vi "Fetch Multi Eval Meas Power Dynamics Results.vi"(8 "error in (no error)":errorcluster, 9 "Result Type (Current)":i32(ring) items=["Current"=0, "Average"=1, "Standard Deviation"=3, "Maximum"=4, "Minimum"=5], 10 "Instance (1)":T2=1, 11 "VISA resource name":refnum<visa-resource-name>) -> (0 "error out":errorcluster, 1 "Results":T1 {"Off Power After" format="%^.3e"; "On Power Peak" format="%^.3e"; "On Power RMS" format="%^.3e"; "Off Power Before" format="%^.3e"}, 2 "Reliability":i32, 3 "VISA resource name out":refnum<visa-resource-name>, 4 "Out Of Tolerance":dbl format="%^.3e")   [LabVIEW 2015, in "Rohde&Schwarz CMXP NR FR2 Measurement.lvlib"]
doc: "Returns the average single value results of the power dynamics measurement.\n\nAttributes:\nRSCMXPNRFR2M_ATTR_FETCH_MULTI_EVAL_MEASUREMENT_POWER_DYNAMICS_AVERAGE_RESULTS\nRSCMXPNRFR2M_ATTR_FETCH_MULTI_EVAL_MEASUREMENT_POWER_DYNAMICS_CURRENT_RESULTS\nRSCMXPNRFR2M_ATTR_FETCH_MULTI_EVAL_MEASUREMENT_POWER_DYNAMICS_MAXIMUM_RESULTS\nRSCMXPNRFR2M_ATTR_FETCH_MULTI_EVAL_MEASUREMENT_POWER_DYNAMICS_MINIMUM_RESULTS\nRSCMXPNRFR2M_ATTR_FETCH_MULTI_EVAL_MEASUREMENT_POWER_DYNAMICS_STANDARD_DEVIATION_RESULTS\n\nRemote-control commands:\nFETCh:NRMMw:MEAS<i>:MEValuation:PDYNamics:AVERage?\nFETCh:NRMMw:MEAS<i>:MEValuation:PDYNamics:CURRent?\nFETCh:NRMMw:MEAS<i>:MEValuation:PDYNamics:MAXimum?\nFETCh:NRMMw:MEAS<i>:MEValuation:PDYNamics:MINimum?\nFETCh:NRMMw:MEAS<i>:MEValuation:PDYNamics:SDEViation?"
uses:
  <instrlib>/Rohde&Schwarz CMXP NR FR2 Measurement/Rohde&Schwarz CMXP NR FR2 Measurement.lvlib
  <instrlib>/Rohde&Schwarz CMXP NR FR2 Measurement/Private/_Instance.ctl
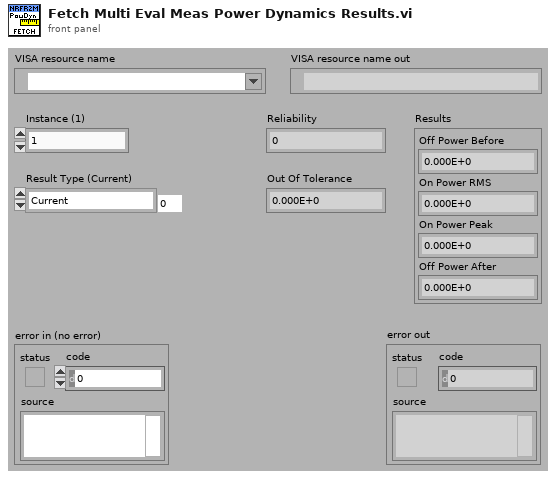
[diagram p1: front panel]
types:
  T1 = cluster{"Off Power Before":dbl, "On Power RMS":dbl, "On Power Peak":dbl, "Off Power After":dbl}
  T2 = typedef "Rohde&Schwarz CMXP NR FR2 Measurement.lvlib/_Instance.ctl" = i32
  T3 = cluster{"Results[0]":dbl, "Results[1]":dbl, "Results[2]":dbl, "Results[3]":dbl}
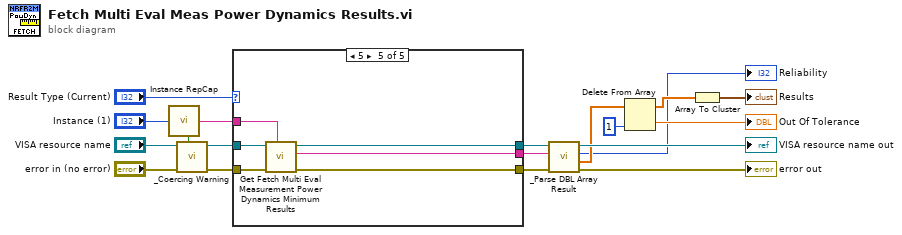
[diagram p0: block diagram]
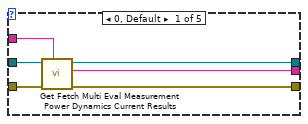
[diagram p2: hidden frame]
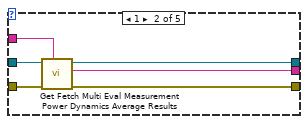
[diagram p3: hidden frame]
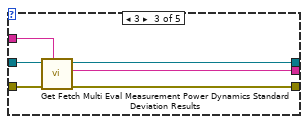
[diagram p4: hidden frame]
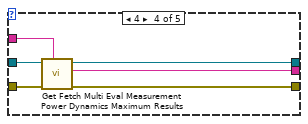
[diagram p5: hidden frame]
diagram:
  n1 = call <instrlib>:"Instance RepCap.vi"("Instance In"="Instance (1)") -> ("In Range?"=w7:bool, "RepCap Identifier Out"=w19:string)  [unwired: 1 in]
  n2 = call <instrlib>:"_Coercing Warning.vi"("In Range?"=w7, "error in (no error)"="error in (no error)", "VISA resource name"="VISA resource name") -> ("error out"=w8:errorcluster, "VISA resource name out"=w9:refnum<visa-resource-name>)  [unwired: 7 in]
  n3 = case shown="5" "Result Type (Current)" {
    tunnel: w19 -> [w25 w31 w37 w43 w49]
    tunnel: w8 -> [w24 w30 w36 w42 w48]
    tunnel: w9 -> [w23 w29 w35 w41 w47]
    tunnel: [w22 w28 w34 w40 w46] -> w18
    tunnel: [w21 w27 w33 w39 w45] -> w17
    tunnel: [w20 w26 w32 w38 w44] -> w16
    frame 0, Default {
      n4 = call "Get Fetch Multi Eval Measurement Power Dynamics Current Results"("Repeated Capabilities"=w25, "error in (no error)"=w24, "instrument handle"=w23) -> ("error out"=w22:errorcluster, "Fetch Multi Eval Measurement Power Dynamics Current Results"=w20:string, "instrument handle out"=w21:refnum<visa-resource-name>)  [unwired: 6 in]
    }
    frame 1 {
      n5 = call "Get Fetch Multi Eval Measurement Power Dynamics Average Results"("Repeated Capabilities"=w31, "error in (no error)"=w30, "instrument handle"=w29) -> ("error out"=w28:errorcluster, "Fetch Multi Eval Measurement Power Dynamics Average Results"=w26:string, "instrument handle out"=w27:refnum<visa-resource-name>)  [unwired: 6 in]
    }
    frame 3 {
      n6 = call "Get Fetch Multi Eval Measurement Power Dynamics Standard Deviation Results"("Repeated Capabilities"=w37, "error in (no error)"=w36, "instrument handle"=w35) -> ("error out"=w34:errorcluster, "Fetch Multi Eval Measurement Power Dynamics Standard Deviation Results"=w32:string, "instrument handle out"=w33:refnum<visa-resource-name>)  [unwired: 6 in]
    }
    frame 4 {
      n7 = call "Get Fetch Multi Eval Measurement Power Dynamics Maximum Results"("Repeated Capabilities"=w43, "error in (no error)"=w42, "instrument handle"=w41) -> ("error out"=w40:errorcluster, "Fetch Multi Eval Measurement Power Dynamics Maximum Results"=w38:string, "instrument handle out"=w39:refnum<visa-resource-name>)  [unwired: 6 in]
    }
    frame 5 {
      n8 = call "Get Fetch Multi Eval Measurement Power Dynamics Minimum Results"("Repeated Capabilities"=w49, "error in (no error)"=w48, "instrument handle"=w47) -> ("error out"=w46:errorcluster, "Fetch Multi Eval Measurement Power Dynamics Minimum Results"=w44:string, "instrument handle out"=w45:refnum<visa-resource-name>)  [unwired: 6 in]
    }
  }
  n9 = call <instrlib>:"_Parse DBL Array Result.vi"("error in (no error)"=w18, "Input String"=w16, "VISA resource name"=w17) -> ("error out"=→"error out":errorcluster, "Results"=w6:dbl[], "Reliability"=→"Reliability":i32, "VISA resource name out"=→"VISA resource name out":refnum<visa-resource-name>)  [unwired: 5 in]
  n10 = Delete From Array(array=w6, index=1) -> (deleted portion=→"Out Of Tolerance":dbl, array with subset deleted=w4:dbl[])  [unwired: 1 in]
  n11 = Array To Cluster(array=w4) -> (cluster=→"Results":T3)
